vi "Sensor_Values.vi"() -> ()   [LabVIEW 2019]
panel:
  in  "Right_Drive_Position":dbl
  in  "Left_Drive_Position":dbl
  in  "Right_Drive_Velocity":dbl
  in  "Left_Drive_Velocity":dbl
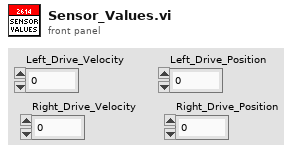
[diagram p1: front panel]
diagram:
